vi "CallbackOnWriteTree.vi"(8 "error in":errorcluster, 11 "node":refnum<data-value>) -> (0 "error out":errorcluster)   [LabVIEW 2013, in "NISE_CEF_Node.lvclass"]
uses:
  Node/NISE_CEF_Node.lvclass
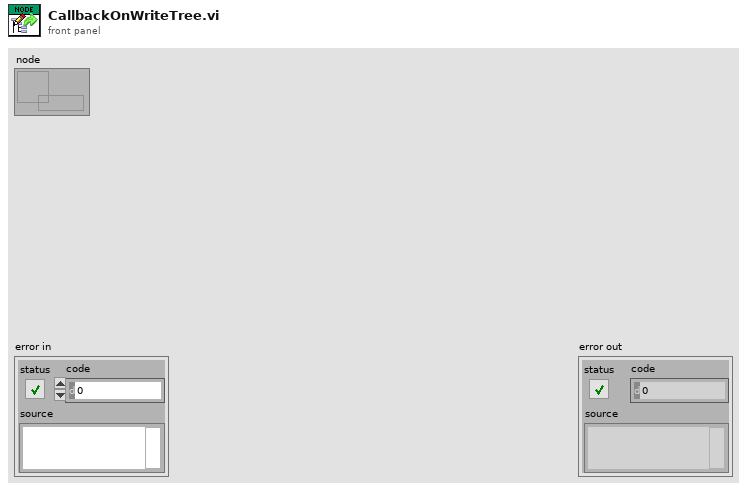
[diagram p1: front panel]
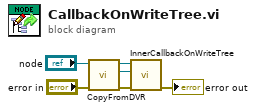
[diagram p0: block diagram]
diagram:
  n1 = call "CopyFromDVR.vi"("error in"="error in", "node in"="node") -> ("error out"=w3:errorcluster, "NISE_CEF_Node out"=w1:refnum<class "NISE_CEF_Node.lvclass">, "node out"=w4:refnum<data-value>)  [unwired: 7 in]
  n2 = call-dynamic "InnerCallbackOnWriteTree.vi"("error in"=w3, "node (for type)"=w1, "node reference"=w4) -> ("error out"=→"error out":errorcluster)  [unwired: 8 in]
